vi "FRCts20_WebMethods_SendNotification.vi"(8 "error in (no error)":errorcluster, 10 "Request Out":T1) -> (0 "error out":errorcluster)   [LabVIEW 2013]
uses:
  Backend/source/VI Source/FRCts20_Backend_API/FRCts20_Backend_API_RequestRoot.ctl
  Backend/source/VI Source/FRCts20_Backend_API/FRCts20_Backend_API_Status.ctl
  Backend/source/VI Source/INI_Accessor/FRCts20_Backend_INI Controller.lvclass
  Backend/source/VI Source/FRCts20_Backend_API/FRCts20_Backend_API.lvlib
panel:
  in  "VI Refnum":refnum<vi>
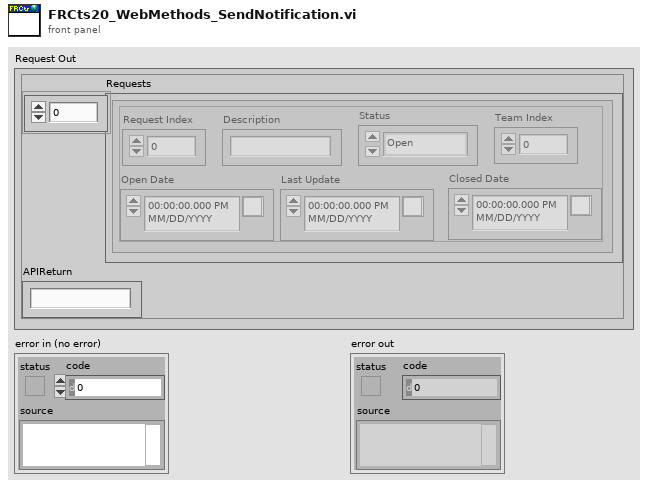
[diagram p1: front panel]
types:
  T1 = typedef "FRCts20_Backend_API.lvlib/FRCts20_Backend_API_RequestRoot.ctl" = cluster{"Requests":cluster{"Request Index":u32, "Description":string, "Status":T2, "Open Date":timestamp, "Last Update":timestamp, "Closed Date":timestamp, "Team Index":u32}[], "APIReturn":string}
  T2 = typedef "FRCts20_Backend_API.lvlib/FRCts20_Backend_API_Status.ctl" = enum16{"Open", "In Work", "Closed"}
  T3 = cluster{"@mailgun domain":string, "API Key":string, "From:":string}
  T4 = cluster{"Request Index":u32, "Description":string, "Status":T2, "Open Date":timestamp, "Last Update":timestamp, "Closed Date":timestamp, "Team Index":u32}[]
  T5 = cluster{"Request Index":u32, "Description":string, "Status":T2, "Open Date":timestamp, "Last Update":timestamp, "Closed Date":timestamp, "Team Index":u32}
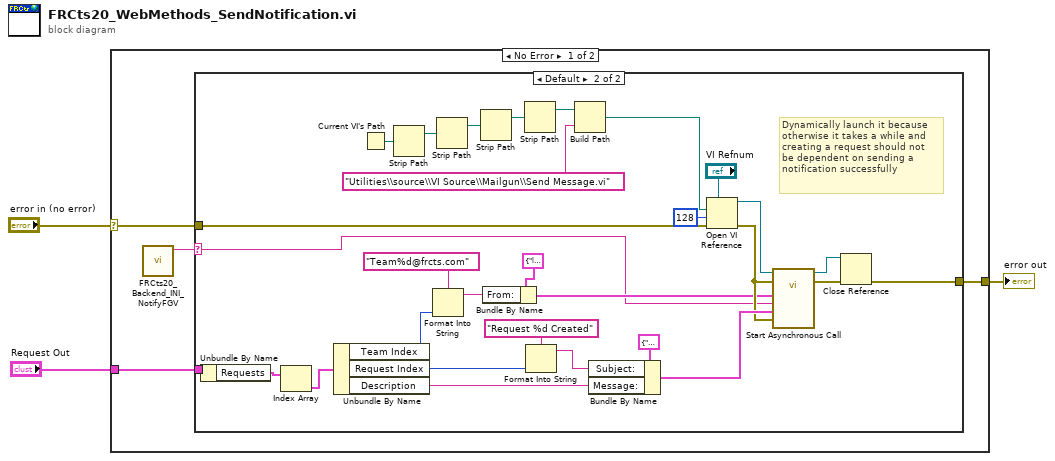
[diagram p0: block diagram]
diagram:
  n1 = case shown="No Error" "error in (no error)" {
    selector: "error in (no error)" -> [w5 w39]
    tunnel: "Request Out" -> [w7 _]
    tunnel: [w6 w39] -> w2
    frame No Error {
      n2 = call "FRCts20_Backend_INI_NotifyFGV.vi"() -> ("Value out"=w4:string)  [unwired: 11 in]
      n3 = case shown="Default" w4 {
        selector: w4 -> [_ w12]
        tunnel: w7 -> [_ w11]
        tunnel: [w8 w16] -> w6
        tunnel: w5 -> [w8 w13]
        frame "" {
          # "Notify no one"
        }
        frame Default {
          # "Dynamically launch it because\notherwise it takes a while and \ncreating a request should not\nbe dependent on sending a\nnotification successfully"
          n4 = Unbundle By Name(w11) -> ("Requests"=w10:T4)
          n5 = Index Array(array=w10) -> (element=w9:T5)  [unwired: 1 in]
          n6 = Unbundle By Name(w9) -> ("Team Index"=w30:u32, "Request Index"=w26:u32, "Description"=w24:string)
          n7 = Current VI's Path() -> (path=w37:path)
          n8 = Strip Path(path=w37) -> (stripped path=w36:path)  [unwired: 1 out]
          n9 = Format Into String(format string="Team%d@frcts.com", w30) -> (resulting string=w28:string)  [unwired: 2 in, 1 out]
          n10 = Strip Path(path=w36) -> (stripped path=w31:path)  [unwired: 1 out]
          n11 = Strip Path(path=w31) -> (stripped path=w32:path)  [unwired: 1 out]
          n12 = Bundle By Name(cluster=T3 {"@mailgun domain"="labview.mailgun.org", "API Key"="api:key-445llei7yq86kemk75g5cvle70ugx-o0", "From:"="christopher.vincent@ni.com"} ("Message Credentials"), "From:"=w28) -> (w15:T3)
          n13 = Strip Path(path=w32) -> (stripped path=w35:path)  [unwired: 1 out]
          n14 = Format Into String(format string="Request %d Created", w26) -> (resulting string=w25:string)  [unwired: 2 in, 1 out]
          n15 = Build Path(base path=w35, name or relative path="Utilities\\source\\VI Source\\Mailgun\\Send Message.vi") -> (appended path=w33:path)
          n16 = Bundle By Name(cluster=cluster{"Subject:":string, "Message:":string} {"Subject:"="Test", "Message:"="Test from VI"} ("Message"), "Subject:"=w25, "Message:"=w24) -> (w21:cluster{"Subject:":string, "Message:":string})
          n17 = Open VI Reference(type specifier VI Refnum (for type only)="VI Refnum", vi path=w33, options=128, error in (no error)=w13) -> (vi reference=w22:refnum<vi>, error out=w19:errorcluster)  [unwired: 2 in]
          n18 = call-by-ref "Start Asynchronous Call"(reference=w22, error in=w19, 8:"error in (no error)"=w19, "Message"=w21, "To:"=w12, "Message Credentials"=w15) -> (reference out=w18:refnum<vi>, error out=w17:errorcluster)  [unwired: 6 in, 2 out]
          n19 = Close Reference(reference=w18, error in (no error)=w17) -> (error out=w16:errorcluster)
        }
      }
    }
    frame Error {
    }
  }
  "error out" <- w2
